vi "ArmManualOverride.vi"(8 "ArmAngleIn":dbl format="%#_13g", 9 "Arm State":T1, 10 "Arm Manual":dbl, 11 "Arm Output":dbl) -> (3 "Final Arm Output":dbl)   [LabVIEW 2014]
uses:
  Typedefs/Arm States.ctl
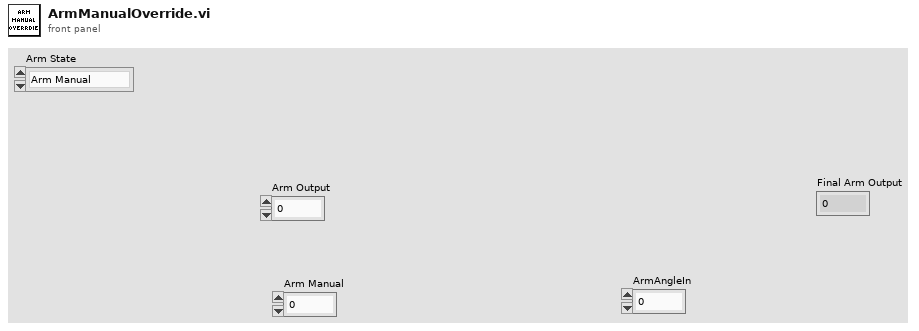
[diagram p1: front panel]
types:
  T1 = typedef "Arm States.ctl" = enum16{"Arm Manual ", "Ground", "Step", "1 Tote", "2 Tote", "3 Tote", "4 Tote", "5 Tote", "6 Tote", "Flip Can", "Grab Can in auto"}
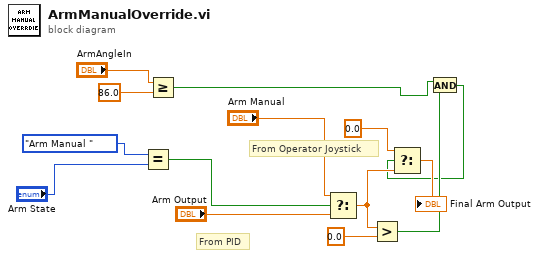
[diagram p0: block diagram]
diagram:
  # "From Operator Joystick"
  # "From PID"
  n1 = Equal?(x=Arm_States."Arm Manual " ("Arm State 2"), y="Arm State") -> (x = y?=w12:bool)
  n2 = Greater Or Equal?(x="ArmAngleIn", y=86.0) -> (x >= y?=w2:bool)
  n3 = Select(t="Arm Manual", s=w12, f="Arm Output") -> (s? t:f=w5:dbl)
  n4 = Greater?(x=w5, y=0.0) -> (0:w3:bool)
  n5 = And(x=w2, y=w3) -> (x .and. y?=w1:bool)
  n6 = Select(t=0.0, s=w1, f=w5) -> (s? t:f=→"Final Arm Output":dbl)
